vi "Create IP.vi"(7 "session":refnum<class "Engine Simulation Session.lvclass">, 8 "error in (no error)":errorcluster, 9 "EST version enum":T1, 10 "Name":string, 11 "Engine Simulation IP in":refnum<class "Engine Simulation IP.lvclass">) -> (0 "error out":errorcluster, 3 "Engine Simulation IP out":refnum<class "Engine Simulation IP.lvclass">)   [LabVIEW 2013, in "Engine Simulation IP.lvclass"]
uses:
  Engine Simulation IP.lvclass
  Bitfile Major Version.ctl
  Engine Simulation Session.lvclass
  IP class private data.ctl
  Engine Simulation IP.lvclass/Engine Simulation IP.ctl
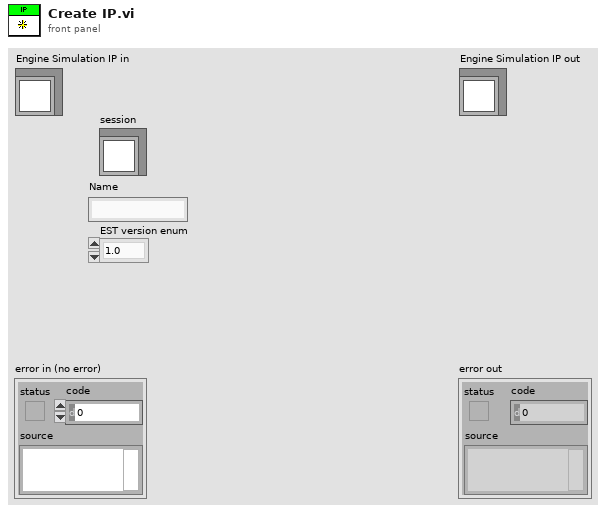
[diagram p1: front panel]
types:
  T1 = typedef "Engine Simulation Session.lvclass/Bitfile Major Version.ctl" = enum16{"1.0", "1.1", "1.2", "1.3"}
  T2 = typedef "Engine Simulation IP.lvclass/IP class private data.ctl" = cluster{"Name":string, "EST version":T1, "session":refnum<class "Engine Simulation Session.lvclass">}
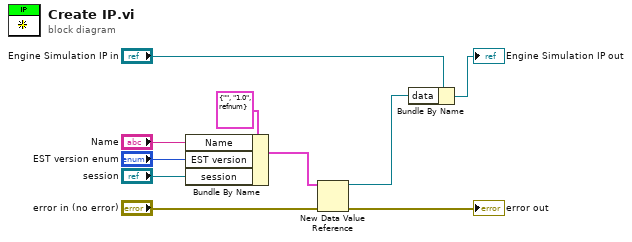
[diagram p0: block diagram]
diagram:
  n1 = Bundle By Name(cluster=T2 {"Name"="", "EST version"=enum."1.0", "session"=refnum} ("data"), "Name"="Name", "EST version"="EST version enum", "session"="session") -> (w5:T2)
  n2 = New Data Value Reference(data value=w5, error in="error in (no error)") -> (data value reference=w2:refnum<data-value>, error out=→"error out":errorcluster)
  n3 = Bundle By Name(cluster="Engine Simulation IP in", "data"=w2) -> (→"Engine Simulation IP out":refnum<class "Engine Simulation IP.lvclass">)
